vi "test Convert Message Definition to Message Configuration.vi"(8 "error in (no error)":errorcluster) -> (0 "error out":errorcluster)   [LabVIEW 2020, in "Create Execution Unit.lvclass"]
uses:
  Create Execution Unit.lvclass
  Shared/Message Definition.ctl
  Shared/Message Type.ctl
  Shared/Terminal Endpoint.ctl
  Shared/Address.ctl
  Shared/Parameter Definition.ctl
  Engine/Custom Device/Message Configuration.ctl
  <vilib>/addons/_JKI Toolkits/VI Tester/TestCase.llb/TestCase.lvclass
  Engine/Implementation/Shared Resources Factory/Shared Resources Factory.lvclass
  Engine/Custom Device/Custom Device.lvlib
  C:/Program Files (x86)/National Instruments/LabVIEW 2020/vi.lib/addons/_JKI Toolkits/VI Tester/TestCase.llb/TestCase.lvclass
panel:
  in  "TestCase in":refnum<class "Create Execution Unit.lvclass">
  out "TestCase out":refnum<class "Create Execution Unit.lvclass">
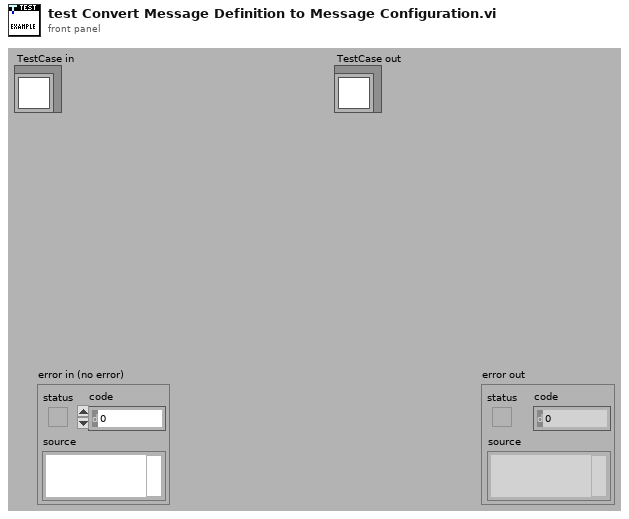
[diagram p1: front panel]
types:
  T1 = typedef "AIM MIL-STD-1553 Engine.lvlib/Custom Device.lvlib/Message Configuration.ctl" = cluster{"Transfer ID":u16, "Transfer Type":enum16{"BC to RT transfer", "RT to BC transfer", "RT to RT transfer"}, "Transmitting RT Address":u8, "Receiving RT Address":u8, "Transmitting RT Sub-address":u8, "Receiving RT Sub-address":u8, "Word Count / Mode Code":u8}
  T2 = typedef "Message Definition.ctl" = cluster{"name":string, "message type":T3, "endpoint Tx":T4, "endpoint Rx":T4, "create timestamp channel":bool, "mode code":u16, "number of words":u16, "parameters":cluster{"name":string, "default value":dbl, "unit":string, "parameter definition":T6}[]}
  T3 = typedef "Message Type.ctl" = string
  T4 = typedef "Terminal Endpoint.ctl" = cluster{"terminal address":T5, "subaddress":T5}
  T5 = typedef "Address.ctl" = u16
  T6 = typedef "Parameter Definition.ctl" = cluster{"start index":i32, "size (bits)":i32, "encoding":enum16{"BNR", "BCD", "Discrete"}, "signed":bool, "multiplier":dbl, "offset":dbl}
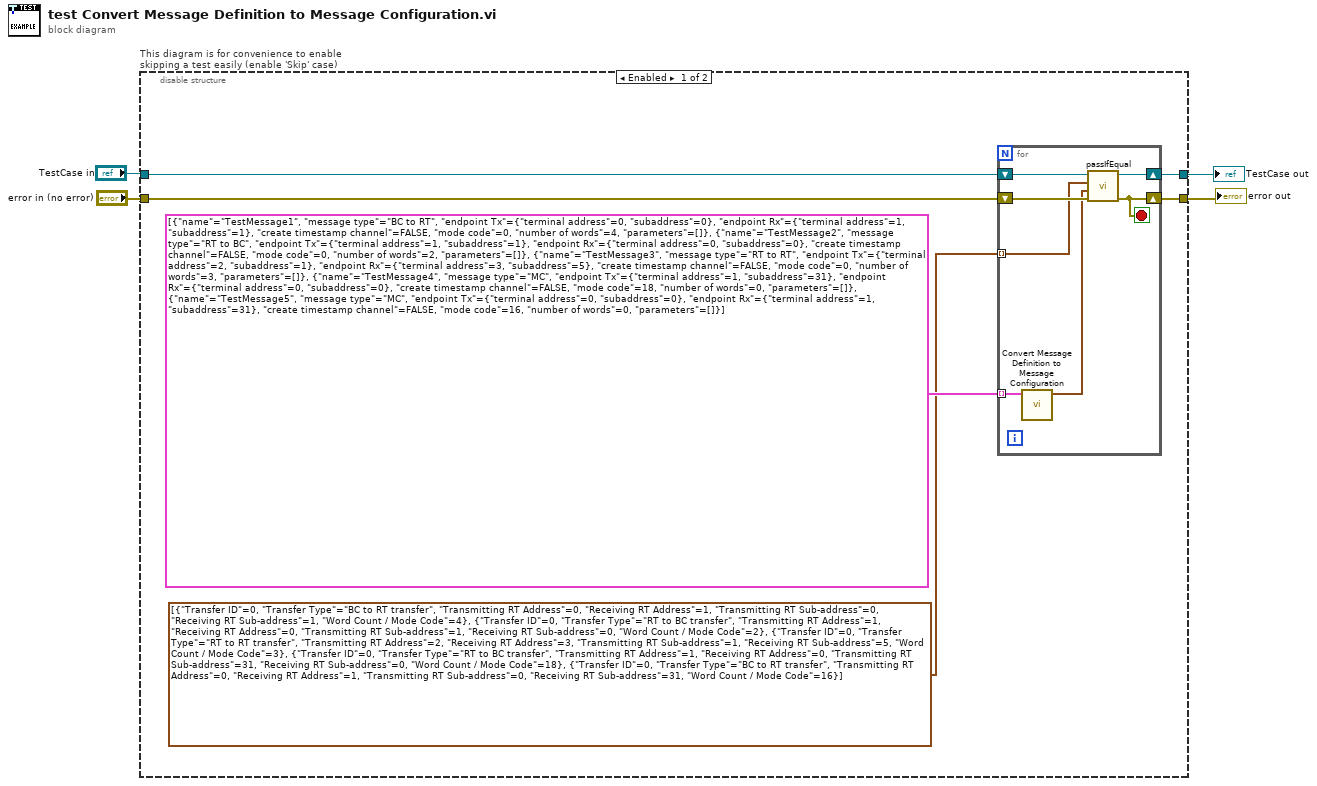
[diagram p0: block diagram]
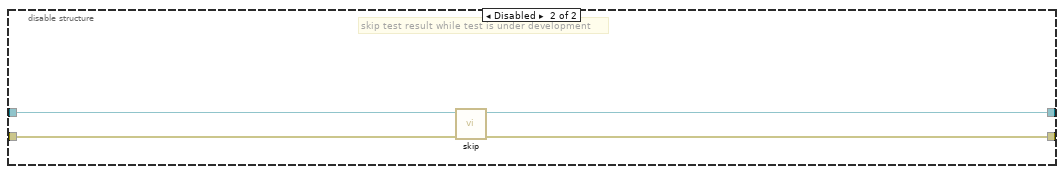
[diagram p2: hidden frame]
diagram:
  n1 = disable-structure "This diagram is for convenience to enable skipping a test easily (enable 'Skip' case)" shown="Enabled" {
    disable-tunnel: "TestCase in" -> [w8 w21]
    disable-tunnel: [w7 w19] -> w1
    disable-tunnel: [w6 w20] -> w3
    disable-tunnel: "error in (no error)" -> [w9 w18]
    frame Enabled {
      n2 = for {
        tunnel: T2[] [{"name"="TestMessage1", "message type"="BC to RT", "endpoint Tx"={"terminal address"=0, "subaddress"=0}, "endpoint Rx"={"terminal address"=1, "subaddress"=1}, "create timestamp channel"=FALSE, "mode code"=0, "number of words"=4, "parameters"=[]}, {"name"="TestMessage2", "message type"="RT to BC", "endpoint Tx"={"terminal address"=1, "subaddress"=1}, "endpoint Rx"={"terminal address"=0, "subaddress"=0}, "create timestamp channel"=FALSE, "mode code"=0, "number of words"=2, "parameters"=[]}, {"name"="TestMessage3", "message type"="RT to RT", "endpoint Tx"={"terminal address"=2, "subaddress"=1}, "endpoint Rx"={"terminal address"=3, "subaddress"=5}, "create timestamp channel"=FALSE, "mode code"=0, "number of words"=3, "parameters"=[]}, {"name"="TestMessage4", "message type"="MC", "endpoint Tx"={"terminal address"=1, "subaddress"=31}, "endpoint Rx"={"terminal address"=0, "subaddress"=0}, "create timestamp channel"=FALSE, "mode code"=18, "number of words"=0, "parameters"=[]}, {"name"="TestMessage5", "message type"="MC", "endpoint Tx"={"terminal address"=0, "subaddress"=0}, "endpoint Rx"={"terminal address"=1, "subaddress"=31}, "create timestamp channel"=FALSE, "mode code"=16, "number of words"=0, "parameters"=[]}] ("Array") -> [w17] mode=indexing
        shift-right: [w11] -> w6
        shift-left: w9 -> [w15]
        shift-right: [w14] -> w7
        shift-left: w8 -> [w16]
        tunnel: T1[] [{"Transfer ID"=0, "Transfer Type"=enum."BC to RT transfer", "Transmitting RT Address"=0, "Receiving RT Address"=1, "Transmitting RT Sub-address"=0, "Receiving RT Sub-address"=1, "Word Count / Mode Code"=4}, {"Transfer ID"=0, "Transfer Type"=enum."RT to BC transfer", "Transmitting RT Address"=1, "Receiving RT Address"=0, "Transmitting RT Sub-address"=1, "Receiving RT Sub-address"=0, "Word Count / Mode Code"=2}, {"Transfer ID"=0, "Transfer Type"=enum."RT to RT transfer", "Transmitting RT Address"=2, "Receiving RT Address"=3, "Transmitting RT Sub-address"=1, "Receiving RT Sub-address"=5, "Word Count / Mode Code"=3}, {"Transfer ID"=0, "Transfer Type"=enum."RT to BC transfer", "Transmitting RT Address"=1, "Receiving RT Address"=0, "Transmitting RT Sub-address"=31, "Receiving RT Sub-address"=0, "Word Count / Mode Code"=18}, {"Transfer ID"=0, "Transfer Type"=enum."BC to RT transfer", "Transmitting RT Address"=0, "Receiving RT Address"=1, "Transmitting RT Sub-address"=0, "Receiving RT Sub-address"=31, "Word Count / Mode Code"=16}] ("Array") -> [w13] mode=indexing
        stop <- w11 stop-if-true
        n3 = call "Convert Message Definition to Message Configuration.vi"("message definition"=w17) -> ("Message Configuration"=w12:T1)  [unwired: 10 in]
        n4 = call-dynamic "passIfEqual.vi"("error in (no error)"=w15, "y"=w12, "x"=w13, "TestCase in"=w16) -> ("error out"=w11:errorcluster, "TestCase out"=w14:refnum<class "Create Execution Unit.lvclass">)  [unwired: 6 in]
      }
    }
    frame Disabled {
      # "skip test result while test is under development"
      n5 = call <vilib>:"skip.vi"("error in (no error)"=w18, "TestCase in"=w21) -> ("error out"=w20:errorcluster, "TestCase out"=w19:refnum<class "Create Execution Unit.lvclass">)  [unwired: 8 in]
    }
  }
  "error out" <- w3
  "TestCase out" <- w1
